vi "LV SciSDK CUSTOM PACKET START.vi"(0 "Custom Packet Name":string, 1 "High Performance":string(combo)="false", 2 "Acq Mode":string(combo)="blocking", 3 "Thread":string(combo)="false", 4 "Handle In":T1, 5 "error in (no error)":errorcluster, 6 "Check Align Word":string(combo)="false", 8 "Timeout":i32=100, 10 "Acq Len":u32=1024, 12 "Threaded Buffer Size":u32=100000) -> (17 "CP Handle Out":cluster{"CP Path":string, "CP Name":string}, 18 "Board Handle Out":T1, 19 "error out":errorcluster)   [LabVIEW 2021, in "SciSDK_Labview.lvlib"]
uses:
  SciSDK_Labview.lvlib
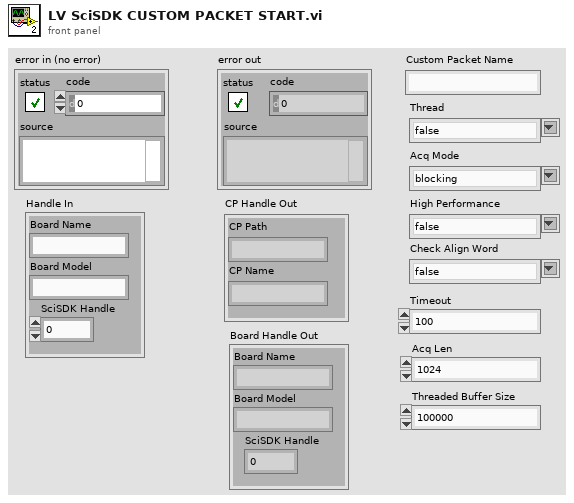
[diagram p1: front panel]
types:
  T1 = cluster{"Board Name":string, "Board Model":string, "SciSDK Handle":u64}
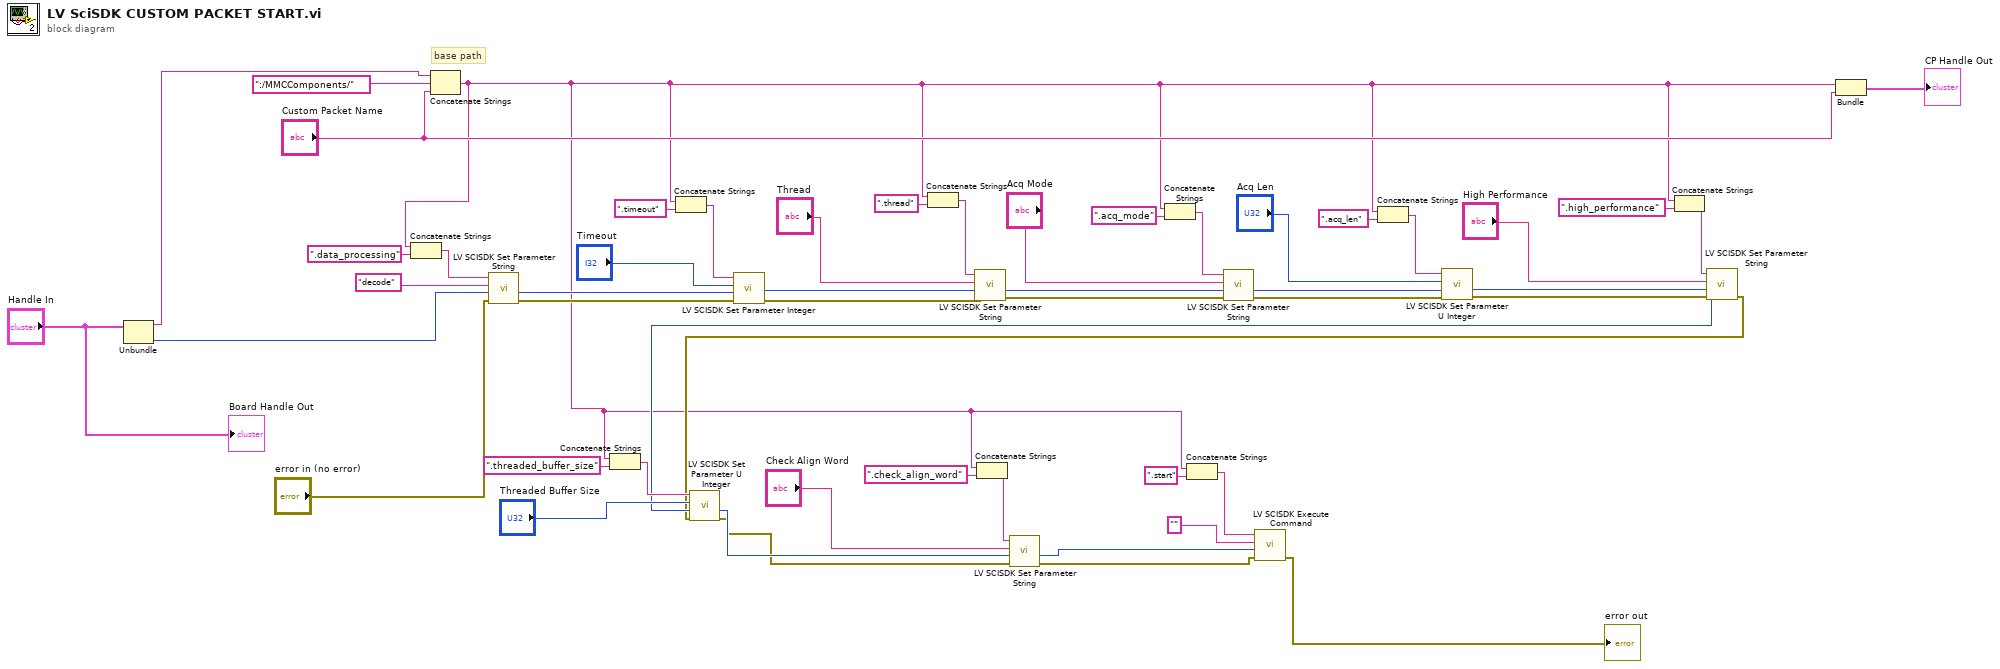
[diagram p0: block diagram]
diagram:
  # "base path"
  n1 = Unbundle("Handle In") -> ("Board Name"=w51:string, "SciSDK Handle"=w46:u64)  [unwired: 1 out]
  n2 = Concatenate Strings(w51, ":/MMCComponents/" ("string"), "Custom Packet Name") -> (w5:string)
  n3 = Concatenate Strings(w5, ".data_processing" ("string")) -> (w48:string)
  n4 = call "LV SCISDK Set Parameter String.vi"("error in (no error)"="error in (no error)", "handle"=w46, "value"="decode", "Path"=w48) -> ("error out"=w32:errorcluster, "handle out"=w43:u64)  [unwired: 5 in, 1 out]
  n5 = Concatenate Strings(w5, ".threaded_buffer_size" ("string")) -> (w18:string)
  n6 = Concatenate Strings(w5, ".timeout" ("string")) -> (w41:string)
  n7 = call "LV SCISDK Set Parameter Integer.vi"("error in (no error)"=w32, "handle"=w43, "value"="Timeout", "Path"=w41) -> ("error out"=w31:errorcluster, "handle out"=w33:u64)  [unwired: 5 in, 1 out]
  n8 = Concatenate Strings(w5, ".thread" ("string")) -> (w39:string)
  n9 = call "LV SCISDK Set Parameter String.vi"("error in (no error)"=w31, "handle"=w33, "value"="Thread", "Path"=w39) -> ("error out"=w30:errorcluster, "handle out"=w34:u64)  [unwired: 5 in, 1 out]
  n10 = Concatenate Strings(w5, ".check_align_word" ("string")) -> (w12:string)
  n11 = Concatenate Strings(w5, ".acq_mode" ("string")) -> (w37:string)
  n12 = Concatenate Strings(w5, ".start" ("string")) -> (w7:string)
  n13 = call "LV SCISDK Set Parameter String.vi"("error in (no error)"=w30, "handle"=w34, "value"="Acq Mode", "Path"=w37) -> ("error out"=w29:errorcluster, "handle out"=w28:u64)  [unwired: 5 in, 1 out]
  n14 = Concatenate Strings(w5, ".acq_len" ("string")) -> (w26:string)
  n15 = call "LV SCISDK Set Parameter U Integer.vi"("error in (no error)"=w29, "handle"=w28, "value"="Acq Len", "Path"=w26) -> ("error out"=w23:errorcluster, "handle out"=w22:u64)  [unwired: 5 in, 1 out]
  n16 = Concatenate Strings(w5, ".high_performance" ("string")) -> (w20:string)
  n17 = call "LV SCISDK Set Parameter String.vi"("error in (no error)"=w23, "handle"=w22, "value"="High Performance", "Path"=w20) -> ("error out"=w15:errorcluster, "handle out"=w16:u64)  [unwired: 5 in, 1 out]
  n18 = call "LV SCISDK Set Parameter U Integer.vi"("error in (no error)"=w15, "handle"=w16, "value"="Threaded Buffer Size", "Path"=w18) -> ("error out"=w10:errorcluster, "handle out"=w11:u64)  [unwired: 5 in, 1 out]
  n19 = call "LV SCISDK Set Parameter String.vi"("error in (no error)"=w10, "handle"=w11, "value"="Check Align Word", "Path"=w12) -> ("error out"=w4:errorcluster, "handle out"=w2:u64)  [unwired: 5 in, 1 out]
  n20 = call "LV SCISDK Execute Command.vi"("error in (no error)"=w4, "handle"=w2, "value"="", "Path"=w7) -> ("error out"=→"error out":errorcluster)  [unwired: 5 in, 2 out]
  n21 = Bundle(w5, "Custom Packet Name"="Custom Packet Name") -> (→"CP Handle Out":cluster{string, "Custom Packet Name":string})  [unwired: 1 in]
  "Board Handle Out" <- "Handle In"
